vi "Emballage_BDD_GVF_chemin_TXT.vi"(6 "Produits_Commandes_en_cours.txt IN":path, 8 "Error in":errorcluster caption="Error in (no error)", 11 "Énum":enum16{"get", "set"}(ring)) -> (0 "Error out":errorcluster, 1 "Produits_Commandes_en_cours.txt OUT":path)   [LabVIEW 2020]
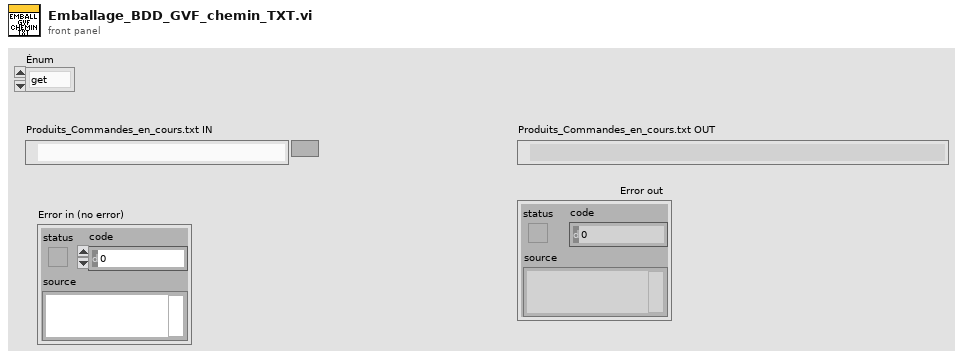
[diagram p1: front panel]
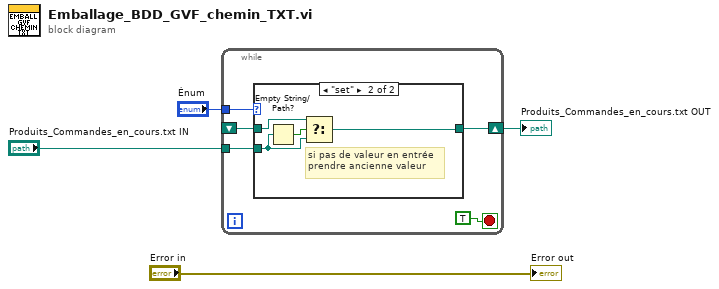
[diagram p0: block diagram]
diagram:
  n1 = while {
    tunnel: "Énum" -> [w8]
    tunnel: "Produits_Commandes_en_cours.txt IN" -> [w5]
    shift-right: [w7] -> w3
    shift-left: _ -> [w6]
    stop <- TRUE stop-if-true
    n2 = case shown="\"set\"" w8 {
      tunnel: [w10 w12] -> w7
      tunnel: w6 -> [w10 w11]
      tunnel: w5 -> [_ w13]
      frame "get", Default {
      }
      frame "set" {
        # "si pas de valeur en entrée \nprendre ancienne valeur"
        n3 = Empty String/Path?(string/path=w13) -> (empty?=w14:bool)
        n4 = Select(t=w11, s=w14, f=w13) -> (s? t:f=w12:path)
      }
    }
  }
  "Produits_Commandes_en_cours.txt OUT" <- w3
  "Error out" <- "Error in"
